vi "Find Object Items by Path.vi"(7 "Item Path":string, 8 "error in (no error)":errorcluster, 10 "Object Offset":i32, 11 "JSON":string) -> (0 "error out":errorcluster, 1 "<JSON>Items":string[](array[string]), 2 "Offsets":i32[](array[numeric]), 3 "Names":string[](array[string]))   [LabVIEW 2015, in "JSONtext.lvlib"]
doc: "Find the JSON items at the JSON Path specified and returns them as an array.\n\nPaths specify an item in a tree of nested Objects, and start with $. Paths may point to multiple items, in the presence either of Arrays, or of multiple specified locations (using a [] form, see example).\n\nExample JSON:\n{\"A\":[{\"C\":123,\"D\":4},{\"C\":567,\"D\":8}],\"B\":\"Hi\",\"E\":true}\nAt path $.A.C are 123 and 567\nAt path $.B (or just B) is \"Hi\"\nAt path $.[B,E] are \"Hi\" and true"
uses:
  JSONtext.lvlib
  support/Unescape JSON string.vi
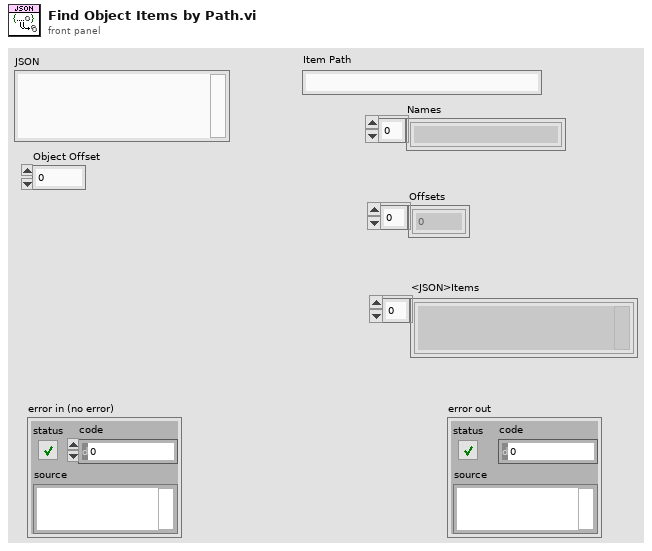
[diagram p1: front panel]
types:
  T1 = typedef "JSONtext.lvlib/Found Items.ctl" = cluster{"Item offset":i32, "Offset past Item":i32, "Name offset":i32, "Offset past Name":i32, "Found":bool, "Item Type":T2, "Item Index":i32}
  T2 = typedef "JSONtext.lvlib/Parsing State.ctl" = enum16{"Parser Error", "Object", "Array", "String", "Number/Other", "Leading Whitespace", "Object end", "Array end", "Value end"}
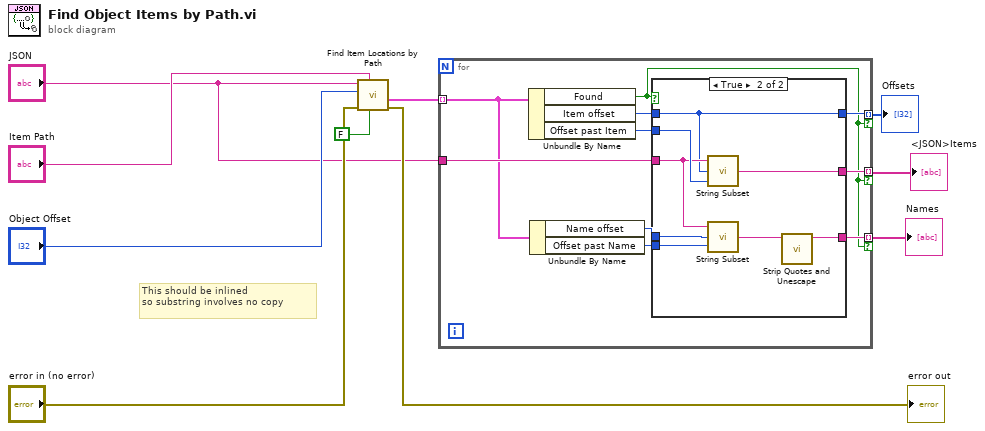
[diagram p0: block diagram]
diagram:
  # "This should be inlined\nso substring involves no copy"
  n1 = call "Find Item Locations by Path.vi"("Only return first found"=FALSE, "Path"="Item Path", "error in (no error)"="error in (no error)", "Object Offset"="Object Offset", "JSON"="JSON") -> ("error out"=→"error out":errorcluster, "Items"=w4:T1[])  [unwired: 5 in]
  n2 = for {
    tunnel: "JSON" -> [w20]
    tunnel: [w19] -> w5 mode=indexing if=w11
    tunnel: w4 -> [w16] mode=indexing
    tunnel: [w13] -> w3 mode=indexing if=w11
    tunnel: [w12] -> w1 mode=indexing if=w11
    n3 = Unbundle By Name(w16) -> ("Found"=w11:bool, "Item offset"=w18:i32, "Offset past Item"=w17:i32)
    n4 = Unbundle By Name(w16) -> ("Name offset"=w14:i32, "Offset past Name"=w15:i32)
    n5 = case shown="True" w11 {
      tunnel: w20 -> [_ w26]
      tunnel: [_ w28] -> w19
      tunnel: w18 -> [_ w21]
      tunnel: w17 -> [_ w27]
      tunnel: w15 -> [_ w25]
      tunnel: w14 -> [_ w24]
      tunnel: [_ w22] -> w13
      tunnel: [_ w21] -> w12
      frame False {
      }
      frame True {
        n6 = call "String Subset.vi"("Offset past End"=w27, "Start offset"=w21, "JSON"=w26) -> ("substring"=w28:string)  [unwired: 2 in]
        n7 = call "String Subset.vi"("Offset past End"=w25, "Start offset"=w24, "JSON"=w26) -> ("substring"=w23:string)  [unwired: 2 in]
        n8 = call "Strip Quotes and Unescape.vi"("String"=w23) -> ("result string"=w22:string)  [unwired: 9 in, 1 out]
      }
    }
  }
  "<JSON>Items" <- w5
  "Names" <- w3
  "Offsets" <- w1
